vi "HR_Zones_Format.vi"(8 "error in (no error)":errorcluster, 11 "wejœcie":T1={"Runer's Data"={"Name"="", "Age"=0}, "HR Max"=0, "Raw Data"={"Time"=[], "Bpm"=[]}, "% HR MAX "=[], "HR Zones "=[], "no of points"=[], "Heart Rate Zone No 2"=[1, 2, 3, 4, 5]}) -> (0 "error out":errorcluster, 3 "wyjœcie":T1={"Runer's Data"={"Name"="", "Age"=0}, "HR Max"=0, "Raw Data"={"Time"=[], "Bpm"=[]}, "% HR MAX "=[], "HR Zones "=[], "no of points"=[], "Heart Rate Zone No 2"=[1, 2, 3, 4, 5]})   [LabVIEW 2024]
uses:
  klaster 4.ctl
  klaster.ctl
  klaster 2.ctl
  f348dc3d-8c6e-4ad5-80a6-e702c0baa233.vi
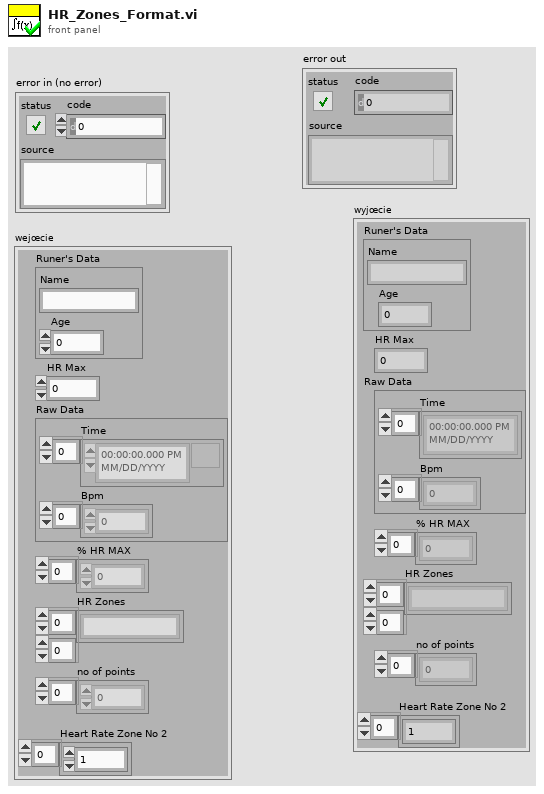
[diagram p1: front panel]
types:
  T1 = typedef "klaster 4.ctl" = cluster{"Runer's Data":T2, "HR Max":i32, "Raw Data":T3, "% HR MAX ":dbl[], "HR Zones ":string[][], "no of points":dbl[], "Heart Rate Zone No 2":i32[]}
  T2 = typedef "klaster.ctl" = cluster{"Name":string, "Age":i32}
  T3 = typedef "klaster 2.ctl" = cluster{"Time":timestamp[], "Bpm":i32[]}
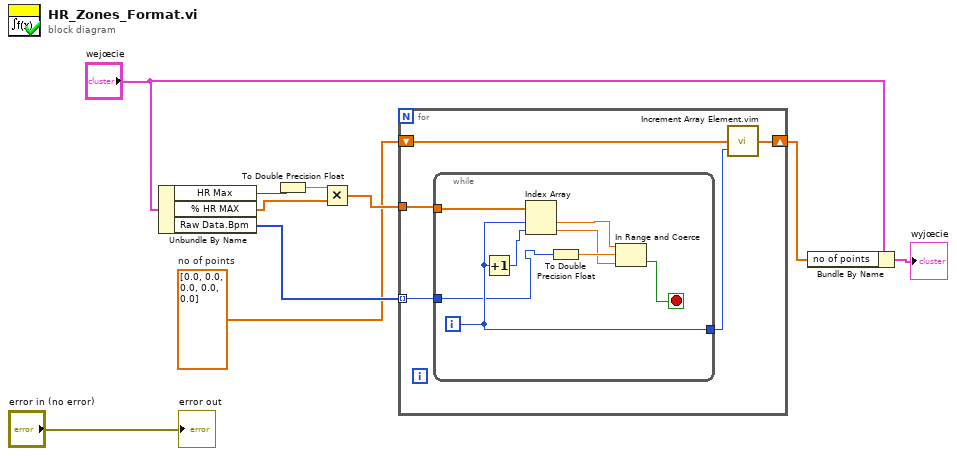
[diagram p0: block diagram]
diagram:
  w2 = dbl[] [0.0, 0.0, 0.0, 0.0, 0.0]  # no of points
  n1 = Unbundle By Name("wejœcie") -> ("HR Max"=w5:i32, "% HR MAX"=w1:dbl[], "Raw Data.Bpm"=w3:i32[])
  n2 = To Double Precision Float(number=w5) -> (double precision float=w4:dbl)
  n3 = Multiply(x=w4, y=w1) -> (x*y=w10:dbl[])
  n4 = for {
    tunnel: w3 -> [w15] mode=indexing
    tunnel: w10 -> [w11]
    shift-right: [w13] -> w9
    shift-left: w2 -> [w14]
    n5 = while {
      tunnel: w11 -> [w18]
      tunnel: w15 -> [w20]
      tunnel: [w22] -> w12
      i -> [w22]
      stop <- w21 stop-if-true
      n6 = Increment(x=w22) -> (x+1=w23:i32)
      n7 = Index Array(array=w18, index #1=w22, index #2=w23) -> (element #1=w16:dbl, element #2=w17:dbl)
      n8 = To Double Precision Float(number=w20) -> (double precision float=w19:dbl)
      n9 = In Range and Coerce(upper limit=w16, x=w19, lower limit=w17) -> (In Range?=w21:bool)  [unwired: 1 out]
    }
    n10 = call "Increment Array Element.vim"("index"=w12, "array in"=w14) -> ("array out"=w13:dbl[])
  }
  n11 = Bundle By Name(cluster="wejœcie", "no of points"=w9) -> (→"wyjœcie":T1)
  "error out" <- "error in (no error)"
